vi "Battery_Model_Pulsed_Current.vi"() -> ()   [LabVIEW 2015]
uses:
  <vilib>/Platform/TimedLoop/XDataNode/timing_clust.ctl
  <vilib>/Platform/TimedLoop/XDataNode/nitl_modes.ctl
  <vilib>/Platform/TimedLoop/XDataNode/wakeup.ctl
  Global 1.vi
  <vilib>/Utility/NIReport.llb/NI_report.lvclass
  <vilib>/platform/TimedLoop/XDataNode/XDataNode.xnode
  <instrlib>/Agilent N6700 Series/Agilent N6700 Series.lvlib
  <vilib>/addons/_office/NI_ReportGenerationToolkit.lvlib
  <vilib>/Platform/TimedLoop/XDataNode/XDNodeRunTimeDep.lvlib
panel:
  in  "Stop":bool
  out "Voltage Graph":dbl[](graph)
  in  "Negative Voltage Limit (0.0 volts) 3":dbl format="%^.3e"
  in  "Priority (1: Voltage) 3":i32(ring) items=["Voltage"=1, "Current"=0]
  in  "Positive Voltage Limit  (5.0 V) 3":dbl=5.0 format="%^.3e"
  in  "Channel Name (1) 3":string="4"
  in  "VISA resource name 3":refnum<visa-resource-name>="USB0::0x0957::0x0F07::MY53002228::INSTR"
  in  "report file path 4":path=path "C:/Users/Tulio/Documents/LabView Projects/Battery Model/Battery_Model_Measurements.xlsx"
  out "Current Graph":dbl[](graph)
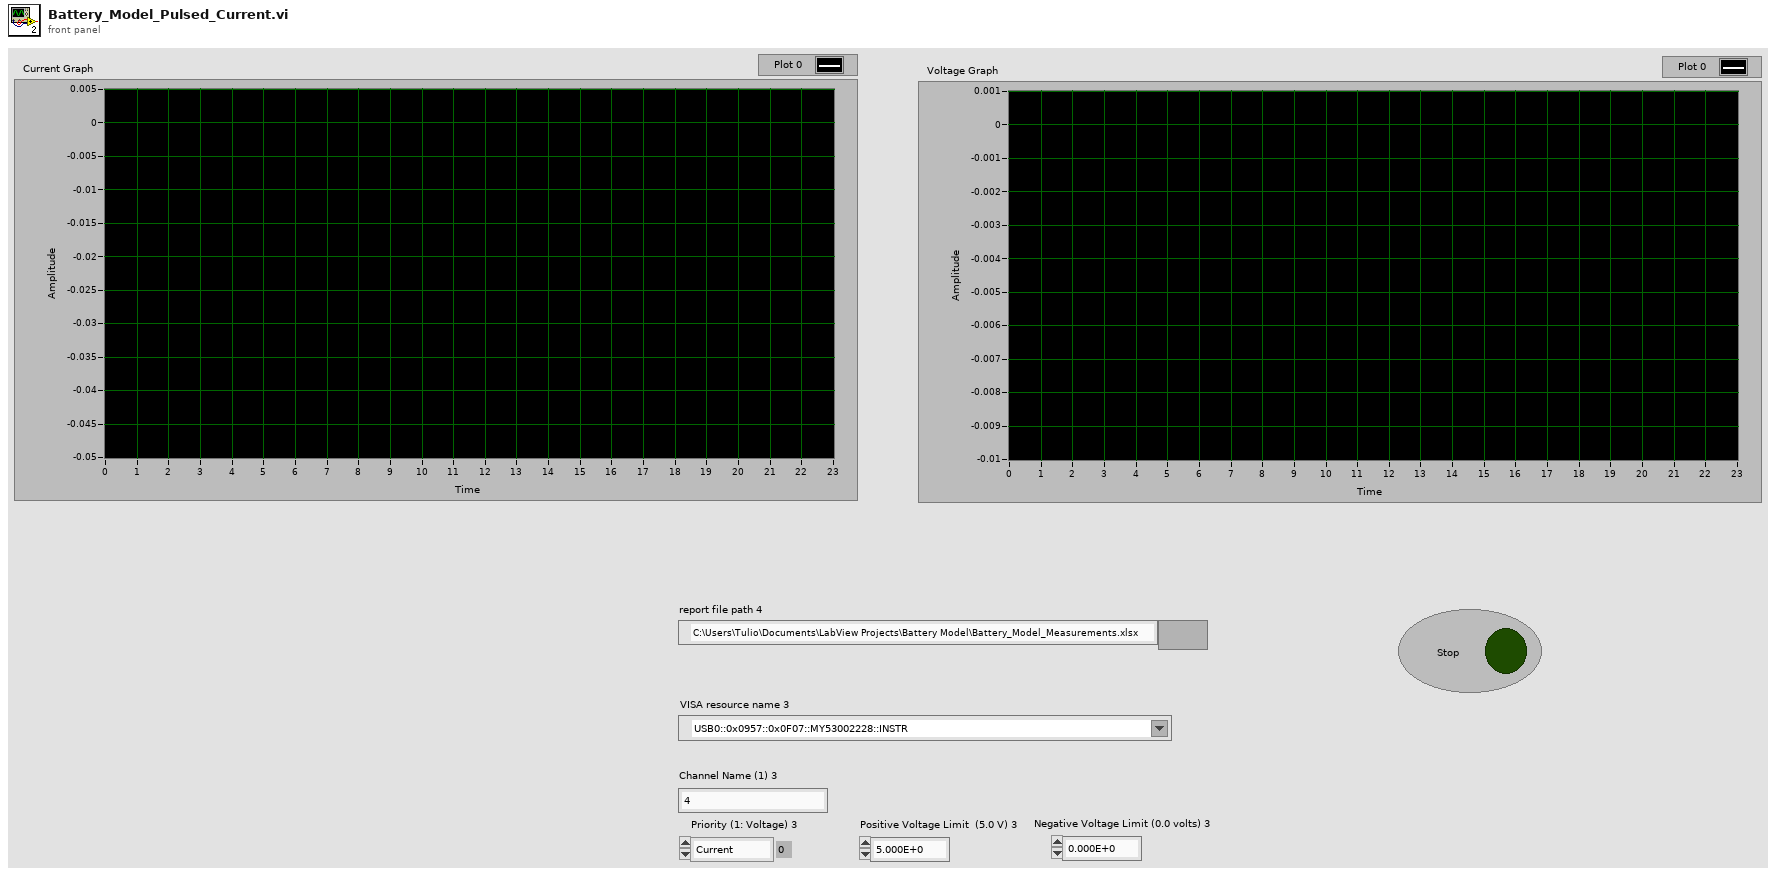
[diagram p1: front panel]
types:
  T1 = enum16{"Standard Report", "HTML", "Word", "Excel"}
  T2 = typedef "XDNodeRunTimeDep.lvlib/timing_clust.ctl" = cluster{"Expected End [f-1]":u64, "Actual End [f-1]":u64, "Finished Late? [f-1]":bool, "Expected End [i-1]":u64, "Actual End [i-1]":u64, "Finished Late? [i-1]":bool, "Expected Start [i]":u64, "Actual Start [i]":u64, "Expected Start [f]":u64, "Actual Start [f]":u64, "Source Name":string, "Structure Name":string, "Period":i64, "Deadline":i64, "Offset":i64, "Start":i64, "Priority":i32, "Timeout":i32, "Mode":T3, "Wakeup Reason":T4, "Error":errorcluster, "Source Type":string, "Secondary Source Type":string, "Global End Time":u64, "Global Start Time":u64, "Frame Duration":u64, "Iteration Duration":u64, "Assigned CPU":i32, "I/O Scan Engine Mode":u32}
  T3 = typedef "XDNodeRunTimeDep.lvlib/nitl_modes.ctl" = enum32{"No Change", "Process missed periods, maintain original phase", "Discard missed periods, maintain original phase", "Process missed periods, ignore original phase", "Discard missed periods, ignore original phase"}
  T4 = typedef "XDNodeRunTimeDep.lvlib/wakeup.ctl" = enum32{"Normal", "Aborted", "Asynchronous wakeup", "Timing source error", "Timed loop error", "Timeout"}
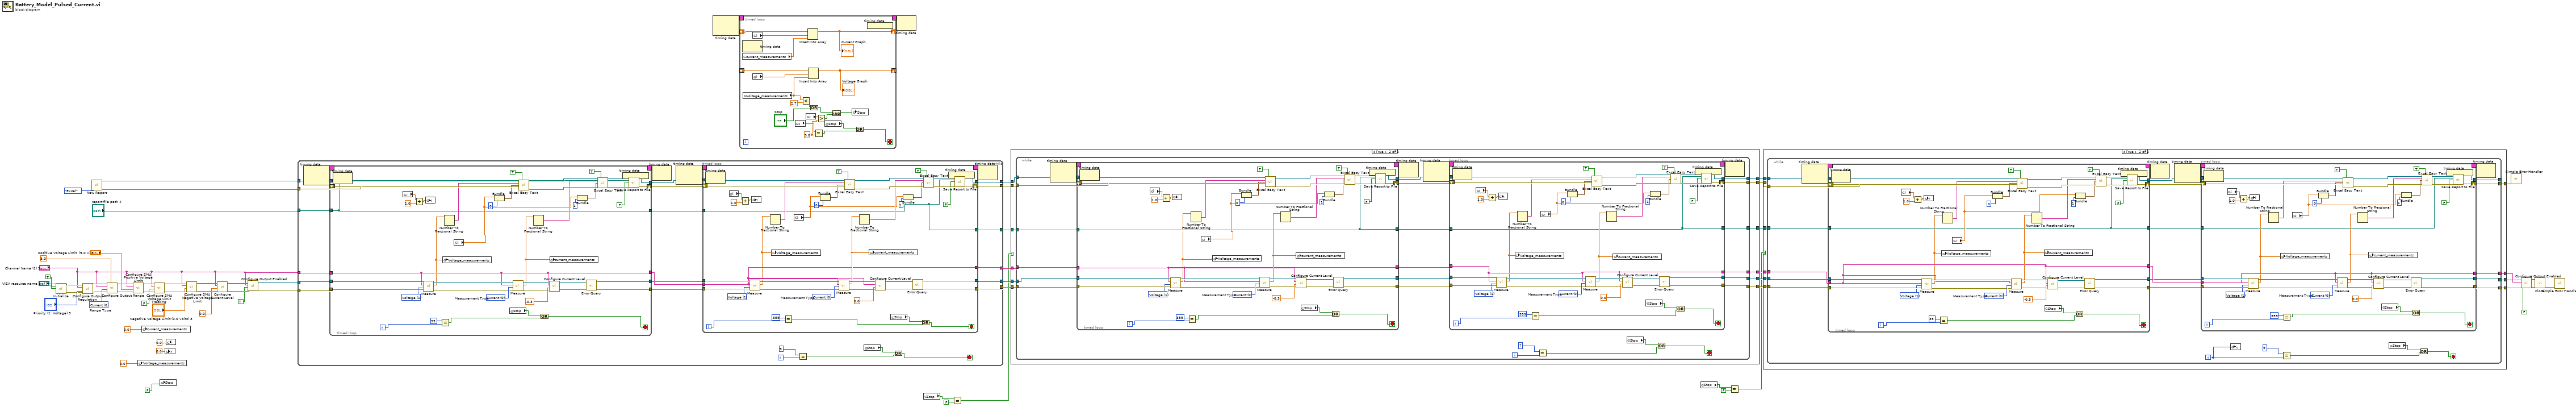
[diagram p0: block diagram]
diagram:
  w49 = TRUE ("Reset? (T: Yes)")
  w48 = 0 items=["Voltage"=1, "Current"=0]  # Range Type
  n1 = call <instrlib>:"Initialize.vi"("VISA resource name"="VISA resource name 3", "ID Query? (T: Yes)"=w49, "Reset? (T: Yes)"=w49) -> ("VISA resource name out"=w38:refnum<visa-resource-name>, "error out"=w37:errorcluster)  [unwired: 11 in]
  n2 = call <instrlib>:"Configure Output Regulation.vi"("VISA resource name"=w38, "Channel Name (1)"="Channel Name (1) 3", "Output Regulation Priority (1: Voltage)"="Priority (1: Voltage) 3", "error in (no error)"=w37) -> ("VISA resource name out"=w50:refnum<visa-resource-name>, "error out"=w51:errorcluster)  [unwired: 10 in]
  n3 = call <vilib>:"New Report.vi"("report type"=T1."Excel") -> ("report out"=w61:refnum<class "NI_report.lvclass">, "error out"=w60:errorcluster)  [unwired: 13 in]
  n4 = call <instrlib>:"Configure Output Range.vi"("Range (0.0)"=3.0, "error in (no error)"=w51, "Range Type (1: Voltage)"=w48, "Channel Name (1)"="Channel Name (1) 3", "VISA resource name"=w50) -> ("error out"=w53:errorcluster, "VISA resource name out"=w52:refnum<visa-resource-name>)  [unwired: 5 in]
  n5 = call <instrlib>:"Configure SMU Positive Voltage Limit.vi"("error in (no error)"=w53, "Positive Voltage Limit (0.0 volts)"="Positive Voltage Limit  (5.0 V) 3", "Channel Name (1)"="Channel Name (1) 3", "VISA resource name"=w52) -> ("error out"=w55:errorcluster, "VISA resource name out"=w54:refnum<visa-resource-name>)  [unwired: 6 in]
  n6 = global write "Global 1.vi" "Voltage_measurements"(0.0 ("Actual_hour")) -> ()
  n7 = global write "Global 1.vi" "current_measurements"(0.0 ("Actual_hour")) -> ()
  n8 = call <instrlib>:"Configure SMU Voltage Limit Tracking.vi"("error in (no error)"=w55, "Enable Voltage Limit Tracking (False)"=FALSE, "Channel Name (1)"="Channel Name (1) 3", "VISA resource name"=w54) -> ("error out"=w42:errorcluster, "VISA resource name out"=w43:refnum<visa-resource-name>)  [unwired: 6 in]
  n9 = global write "Global 1.vi" "Stop"(FALSE ("Stop")) -> ()
  n10 = global write "Global 1.vi" "x"(0.0 ("x")) -> ()
  n11 = global write "Global 1.vi" "i"(0.0 ("Actual_hour")) -> ()
  n12 = call <instrlib>:"Configure SMU Negative Voltage Limit.vi"("error in (no error)"=w42, "Negative Voltage Limit (0.0 volts)"="Negative Voltage Limit (0.0 volts) 3", "Channel Name (1)"="Channel Name (1) 3", "VISA resource name"=w43) -> ("error out"=w39:errorcluster, "VISA resource name out"=w40:refnum<visa-resource-name>)  [unwired: 6 in]
  n13 = call <instrlib>:"Configure Current Level.vi"("error in (no error)"=w39, "Level  (0.0 A)"=0.0, "Channel Name (1)"="Channel Name (1) 3", "VISA resource name"=w40) -> ("error out"=w58:errorcluster, "VISA resource name out"=w59:refnum<visa-resource-name>)  [unwired: 6 in]
  n14 = call <instrlib>:"Configure Output Enabled.vi"("error in (no error)"=w58, "Enable Output (False)"=TRUE, "Channel Name (1)"="Channel Name (1) 3", "VISA resource name"=w59) -> ("error out"=w30:errorcluster, "VISA resource name out"=w31:refnum<visa-resource-name>)  [unwired: 6 in]
  n15 = while {
    tunnel: w31 -> [w89]
    tunnel: w30 -> [w88]
    tunnel: [w68] -> w25
    tunnel: [w70] -> w24
    tunnel: [w72] -> w23
    tunnel: w61 -> [w91]
    tunnel: w60 -> [w90]
    tunnel: "Channel Name (1) 3" -> [w73]
    tunnel: [w78] -> w22
    tunnel: [w77] -> w21
    tunnel: "report file path 4" -> [w76]
    tunnel: [w74] -> w10
    i -> [w80]
    stop <- w66 stop-if-true
    n16 = node-c288() -> (w87:T2)  [unwired: 2 in]
    n17 = timed-loop {
      timing: w87 -> [_]
      timing-out: [_] -> w86
      tunnel: w91 -> [w180]
      tunnel: w73 -> [w143]
      shift-right: [w168] -> w82
      shift-left: w90 -> [w179]
      tunnel: [w148] -> w83
      tunnel: [w143] -> w81
      tunnel: [w144] -> _
      tunnel: w76 -> [w144]
      tunnel: [w144] -> w75
      tunnel: w89 -> [w164]
      tunnel: [w158] -> w71
      tunnel: w88 -> [w163]
      tunnel: [w157] -> w69
      i -> [w146]
      stop <- w139 stop-if-true
      w162 = 1 items=["Current", "Voltage", "Power"] ("Measurement Type (1: Voltage)")
      w181 = 0 items=["Voltage"=1, "Current"=0]  # Measurement Type
      n18 = node-c288() -> ()  [unwired: 1 in, 1 out]
      n19 = global read "Global 1.vi" "i"() -> (w151:dbl)
      n20 = Add(x=w151, y=1.0) -> (x+y=w152:dbl)
      n21 = call <instrlib>:"Measure.vi"("error in (no error)"=w163, "Measurement Type (1: Voltage)"=w162, "Channel Name (1)"=w143, "VISA resource name"=w164) -> ("error out"=w166:errorcluster, "Measurement"=w142:dbl, "VISA resource name out"=w165:refnum<visa-resource-name>)  [unwired: 5 in]
      n22 = global write "Global 1.vi" "i"(w152) -> ()
      n23 = Equal?(x=35, y=w146) -> (x = y?=w141:bool)
      n24 = global write "Global 1.vi" "Voltage_measurements"(w142) -> ()
      n25 = Number To Fractional String(number=w142) -> (F-format string=w161:string)  [unwired: 3 in]
      n26 = global read "Global 1.vi" "i"() -> (w147:dbl)
      n27 = Bundle("i"=w147, "offset (0)"=0) -> (w178:cluster{"i":dbl, "offset (0)":i32})  [unwired: 1 in]
      n28 = global read "Global 1.vi" "Stop"() -> (w140:bool)
      n29 = call <instrlib>:"Measure.vi"("error in (no error)"=w166, "Measurement Type (1: Voltage)"=w181, "Channel Name (1)"=w143, "VISA resource name"=w165) -> ("error out"=w153:errorcluster, "Measurement"=w149:dbl, "VISA resource name out"=w154:refnum<visa-resource-name>)  [unwired: 5 in]
      n30 = call <vilib>:"Excel Easy Text.vi"("report in"=w180, "border? (F)"=TRUE, "text"=w161, "start (-1, -1)"=w178, "error in (no error)"=w179) -> ("report out"=w175:refnum<class "NI_report.lvclass">, "error out"=w176:errorcluster)  [unwired: 6 in, 3 out]
      n31 = Number To Fractional String(number=w149) -> (F-format string=w172:string)  [unwired: 3 in]
      n32 = Or(x=w140, y=w141) -> (x .or. y?=w139:bool)
      n33 = call <instrlib>:"Configure Current Level.vi"("error in (no error)"=w153, "Level  (0.0 A)"=-0.3, "Channel Name (1)"=w143, "VISA resource name"=w154) -> ("error out"=w155:errorcluster, "VISA resource name out"=w156:refnum<visa-resource-name>)  [unwired: 6 in]
      n34 = global write "Global 1.vi" "current_measurements"(w149) -> ()
      n35 = Bundle("i"=w147, "offset (0)"=1) -> (w173:cluster{"i":dbl, "offset (0)":i32})  [unwired: 1 in]
      n36 = call <instrlib>:"Error Query.vi"("VISA resource name"=w156, "error in (no error)"=w155) -> ("VISA resource name out"=w158:refnum<visa-resource-name>, "error out"=w157:errorcluster)  [unwired: 10 in, 2 out]
      n37 = call <vilib>:"Excel Easy Text.vi"("report in"=w175, "border? (F)"=TRUE, "text"=w172, "start (-1, -1)"=w173, "error in (no error)"=w176) -> ("report out"=w170:refnum<class "NI_report.lvclass">, "error out"=w169:errorcluster)  [unwired: 6 in, 3 out]
      n38 = node-c288() -> ()  [unwired: 1 out]
      n39 = call-dynamic "Save Report to File.vi"("report in"=w170, "report file path"=w144, "prompt to replace? (F)"=FALSE, "error in (no error)"=w169) -> ("report out"=w148:refnum<class "NI_report.lvclass">, "error out"=w168:errorcluster)  [unwired: 10 in]
    }
    n40 = node-c288(w86) -> ()  [unwired: 1 out]
    n41 = node-c288() -> (w85:T2)  [unwired: 2 in]
    n42 = timed-loop {
      timing: w85 -> [_]
      timing-out: [_] -> w84
      tunnel: w83 -> [w133]
      tunnel: w81 -> [w96]
      shift-right: [w121] -> w78
      shift-left: w82 -> [w132]
      tunnel: [w98] -> w77
      tunnel: w75 -> [w97]
      tunnel: [w97] -> w74
      tunnel: [w96] -> w72
      tunnel: w71 -> [w117]
      tunnel: [w111] -> w70
      tunnel: w69 -> [w116]
      tunnel: [w110] -> w68
      i -> [w100]
      stop <- w92 stop-if-true
      w115 = 1 items=["Current", "Voltage", "Power"] ("Measurement Type (1: Voltage)")
      w134 = 0 items=["Voltage"=1, "Current"=0]  # Measurement Type
      n43 = node-c288() -> ()  [unwired: 1 in, 1 out]
      n44 = global read "Global 1.vi" "i"() -> (w104:dbl)
      n45 = Add(x=w104, y=1.0) -> (x+y=w105:dbl)
      n46 = call <instrlib>:"Measure.vi"("error in (no error)"=w116, "Measurement Type (1: Voltage)"=w115, "Channel Name (1)"=w96, "VISA resource name"=w117) -> ("error out"=w119:errorcluster, "Measurement"=w95:dbl, "VISA resource name out"=w118:refnum<visa-resource-name>)  [unwired: 5 in]
      n47 = global write "Global 1.vi" "i"(w105) -> ()
      n48 = Number To Fractional String(number=w95) -> (F-format string=w114:string)  [unwired: 3 in]
      n49 = global write "Global 1.vi" "Voltage_measurements"(w95) -> ()
      n50 = Equal?(x=359, y=w100) -> (x = y?=w93:bool)
      n51 = global read "Global 1.vi" "i"() -> (w102:dbl)
      n52 = Bundle("i"=w102, "offset (0)"=0) -> (w131:cluster{"i":dbl, "offset (0)":i32})  [unwired: 1 in]
      n53 = call <instrlib>:"Measure.vi"("error in (no error)"=w119, "Measurement Type (1: Voltage)"=w134, "Channel Name (1)"=w96, "VISA resource name"=w118) -> ("error out"=w106:errorcluster, "Measurement"=w101:dbl, "VISA resource name out"=w107:refnum<visa-resource-name>)  [unwired: 5 in]
      n54 = call <vilib>:"Excel Easy Text.vi"("report in"=w133, "border? (F)"=TRUE, "text"=w114, "start (-1, -1)"=w131, "error in (no error)"=w132) -> ("report out"=w128:refnum<class "NI_report.lvclass">, "error out"=w129:errorcluster)  [unwired: 6 in, 3 out]
      n55 = Number To Fractional String(number=w101) -> (F-format string=w125:string)  [unwired: 3 in]
      n56 = global write "Global 1.vi" "current_measurements"(w101) -> ()
      n57 = call <instrlib>:"Configure Current Level.vi"("error in (no error)"=w106, "Level  (0.0 A)"=0.0, "Channel Name (1)"=w96, "VISA resource name"=w107) -> ("error out"=w108:errorcluster, "VISA resource name out"=w109:refnum<visa-resource-name>)  [unwired: 6 in]
      n58 = global read "Global 1.vi" "Stop"() -> (w94:bool)
      n59 = Bundle("i"=w102, "offset (0)"=1) -> (w126:cluster{"i":dbl, "offset (0)":i32})  [unwired: 1 in]
      n60 = call <instrlib>:"Error Query.vi"("VISA resource name"=w109, "error in (no error)"=w108) -> ("VISA resource name out"=w111:refnum<visa-resource-name>, "error out"=w110:errorcluster)  [unwired: 10 in, 2 out]
      n61 = Or(x=w94, y=w93) -> (x .or. y?=w92:bool)
      n62 = call <vilib>:"Excel Easy Text.vi"("report in"=w128, "border? (F)"=TRUE, "text"=w125, "start (-1, -1)"=w126, "error in (no error)"=w129) -> ("report out"=w123:refnum<class "NI_report.lvclass">, "error out"=w122:errorcluster)  [unwired: 6 in, 3 out]
      n63 = node-c288() -> ()  [unwired: 1 out]
      n64 = call-dynamic "Save Report to File.vi"("report in"=w123, "report file path"=w97, "prompt to replace? (F)"=FALSE, "error in (no error)"=w122) -> ("report out"=w98:refnum<class "NI_report.lvclass">, "error out"=w121:errorcluster)  [unwired: 10 in]
    }
    n65 = Equal?(x=9, y=w80) -> (x = y?=w65:bool)
    n66 = global read "Global 1.vi" "Stop"() -> (w67:bool)
    n67 = Or(x=w67, y=w65) -> (x .or. y?=w66:bool)
    n68 = node-c288(w84) -> ()  [unwired: 1 out]
  }
  n69 = node-c288() -> (w64:T2)  [unwired: 2 in]
  n70 = timed-loop {
    timing: w64 -> [_]
    timing-out: [_] -> w63
    shift-right: [w204] -> _
    shift-left: _ -> [w205]
    shift-right: [w199] -> _
    shift-left: _ -> [w198]
    stop <- w195 stop-if-true
    w186 = 9.0 ("y")
    n71 = node-c288() -> ()  [unwired: 1 in, 1 out]
    n72 = global read "Global 1.vi" "current_measurements"() -> (w202:dbl)
    n73 = global read "Global 1.vi" "Voltage_measurements"() -> (w191:dbl)
    n74 = global read "Global 1.vi" "i"() -> (w203:dbl)
    n75 = global read "Global 1.vi" "i"() -> (w200:dbl)
    n76 = global read "Global 1.vi" "x"() -> (w201:dbl)
    n77 = Less?(x=w191, y=2.7) -> (x < y?=w193:bool)
    n78 = global read "Global 1.vi" "i"() -> (w187:dbl)
    n79 = Insert Into Array(array=w205, index=w203, new element=w202) -> (w204:dbl[])
    "Current Graph" <- w204
    n80 = Insert Into Array(array=w198, index=w200, new element=w191) -> (w199:dbl[])
    "Voltage Graph" <- w199
    n81 = Or(x=w193, y="Stop") -> (x .or. y?=w189:bool)
    n82 = Equal?(x=w201, y=w186) -> (x = y?=w196:bool)
    n83 = Greater?(x=w187, y=w186) -> (0:w188:bool)
    n84 = global read "Global 1.vi" "Stop"() -> (w197:bool)
    n85 = And(x=w189, y=w188) -> (x .and. y?=w190:bool)
    n86 = global write "Global 1.vi" "Stop"(w190) -> ()
    n87 = Or(x=w197, y=w196) -> (x .or. y?=w195:bool)
    n88 = node-c288() -> ()  [unwired: 1 out]
  }
  n89 = node-c288(w63) -> ()  [unwired: 1 out]
  n90 = global read "Global 1.vi" "Stop"() -> (w5:bool)
  n91 = Equal?(x=w5, y=FALSE) -> (x = y?=w6:bool)
  n92 = case shown="True" w6 {
    tunnel: w25 -> [w208 w225]
    tunnel: w24 -> [w209 w224]
    tunnel: w23 -> [w210 w223]
    tunnel: w22 -> [w212 w222]
    tunnel: w21 -> [w213 w221]
    tunnel: [w208 w220] -> w20
    tunnel: [w209 w219] -> w19
    tunnel: [w210 w218] -> w18
    tunnel: [w212 w217] -> w17
    tunnel: [w213 w216] -> w16
    tunnel: w10 -> [w211 w215]
    tunnel: [w211 w214] -> w9
    frame False {
    }
    frame True {
      n93 = while {
        tunnel: w224 -> [w250]
        tunnel: [w230] -> w220
        tunnel: [w231] -> w219
        tunnel: [w233] -> w218
        tunnel: w221 -> [w252]
        tunnel: w222 -> [w251]
        tunnel: w223 -> [w240]
        tunnel: [w239] -> w217
        tunnel: w225 -> [w238]
        tunnel: [w237] -> w216
        tunnel: w215 -> [w236]
        tunnel: [w234] -> w214
        i -> [w242]
        stop <- w227 stop-if-true
        n94 = node-c288() -> (w249:T2)  [unwired: 2 in]
        n95 = timed-loop {
          timing: w249 -> [_]
          timing-out: [_] -> w248
          tunnel: w252 -> [w341]
          tunnel: w240 -> [w308]
          shift-right: [w329] -> w244
          shift-left: w251 -> [w340]
          tunnel: [w309] -> w245
          tunnel: [w308] -> w243
          tunnel: w236 -> [w304]
          tunnel: [w304] -> w235
          tunnel: w250 -> [w325]
          tunnel: [w319] -> w229
          tunnel: w238 -> [w324]
          tunnel: [w318] -> w232
          i -> [w306]
          stop <- w300 stop-if-true
          w323 = 1 items=["Current", "Voltage", "Power"] ("Measurement Type (1: Voltage)")
          w342 = 0 items=["Voltage"=1, "Current"=0]  # Measurement Type
          n96 = node-c288() -> ()  [unwired: 1 in, 1 out]
          n97 = global read "Global 1.vi" "i"() -> (w312:dbl)
          n98 = Add(x=w312, y=1.0) -> (x+y=w313:dbl)
          n99 = call <instrlib>:"Measure.vi"("error in (no error)"=w324, "Measurement Type (1: Voltage)"=w323, "Channel Name (1)"=w308, "VISA resource name"=w325) -> ("error out"=w327:errorcluster, "Measurement"=w303:dbl, "VISA resource name out"=w326:refnum<visa-resource-name>)  [unwired: 5 in]
          n100 = global write "Global 1.vi" "i"(w313) -> ()
          n101 = Equal?(x=359, y=w306) -> (x = y?=w301:bool)
          n102 = Number To Fractional String(number=w303) -> (F-format string=w322:string)  [unwired: 3 in]
          n103 = global read "Global 1.vi" "i"() -> (w307:dbl)
          n104 = global write "Global 1.vi" "Voltage_measurements"(w303) -> ()
          n105 = Bundle("i"=w307, "offset (0)"=0) -> (w339:cluster{"i":dbl, "offset (0)":i32})  [unwired: 1 in]
          n106 = call <instrlib>:"Measure.vi"("error in (no error)"=w327, "Measurement Type (1: Voltage)"=w342, "Channel Name (1)"=w308, "VISA resource name"=w326) -> ("error out"=w314:errorcluster, "Measurement"=w310:dbl, "VISA resource name out"=w315:refnum<visa-resource-name>)  [unwired: 5 in]
          n107 = call <vilib>:"Excel Easy Text.vi"("report in"=w341, "border? (F)"=TRUE, "text"=w322, "start (-1, -1)"=w339, "error in (no error)"=w340) -> ("report out"=w336:refnum<class "NI_report.lvclass">, "error out"=w337:errorcluster)  [unwired: 6 in, 3 out]
          n108 = Number To Fractional String(number=w310) -> (F-format string=w333:string)  [unwired: 3 in]
          n109 = global write "Global 1.vi" "current_measurements"(w310) -> ()
          n110 = call <instrlib>:"Configure Current Level.vi"("error in (no error)"=w314, "Level  (0.0 A)"=-0.3, "Channel Name (1)"=w308, "VISA resource name"=w315) -> ("error out"=w316:errorcluster, "VISA resource name out"=w317:refnum<visa-resource-name>)  [unwired: 6 in]
          n111 = global read "Global 1.vi" "Stop"() -> (w302:bool)
          n112 = Bundle("i"=w307, "offset (0)"=1) -> (w334:cluster{"i":dbl, "offset (0)":i32})  [unwired: 1 in]
          n113 = Or(x=w302, y=w301) -> (x .or. y?=w300:bool)
          n114 = call <instrlib>:"Error Query.vi"("VISA resource name"=w317, "error in (no error)"=w316) -> ("VISA resource name out"=w319:refnum<visa-resource-name>, "error out"=w318:errorcluster)  [unwired: 10 in, 2 out]
          n115 = call <vilib>:"Excel Easy Text.vi"("report in"=w336, "border? (F)"=TRUE, "text"=w333, "start (-1, -1)"=w334, "error in (no error)"=w337) -> ("report out"=w331:refnum<class "NI_report.lvclass">, "error out"=w330:errorcluster)  [unwired: 6 in, 3 out]
          n116 = node-c288() -> ()  [unwired: 1 out]
          n117 = call-dynamic "Save Report to File.vi"("report in"=w331, "report file path"=w304, "prompt to replace? (F)"=FALSE, "error in (no error)"=w330) -> ("report out"=w309:refnum<class "NI_report.lvclass">, "error out"=w329:errorcluster)  [unwired: 10 in]
        }
        n118 = node-c288(w248) -> ()  [unwired: 1 out]
        n119 = node-c288() -> (w247:T2)  [unwired: 2 in]
        n120 = timed-loop {
          timing: w247 -> [_]
          timing-out: [_] -> w246
          tunnel: w245 -> [w294]
          tunnel: w243 -> [w257]
          shift-right: [w282] -> w239
          shift-left: w244 -> [w293]
          tunnel: [w259] -> w237
          tunnel: w235 -> [w258]
          tunnel: [w258] -> w234
          tunnel: [w257] -> w233
          tunnel: w232 -> [w277]
          tunnel: [w271] -> w230
          tunnel: w229 -> [w278]
          tunnel: [w272] -> w231
          i -> [w261]
          stop <- w253 stop-if-true
          w276 = 1 items=["Current", "Voltage", "Power"] ("Measurement Type (1: Voltage)")
          w295 = 0 items=["Voltage"=1, "Current"=0]  # Measurement Type
          n121 = node-c288() -> ()  [unwired: 1 in, 1 out]
          n122 = global read "Global 1.vi" "i"() -> (w265:dbl)
          n123 = Add(x=w265, y=1.0) -> (x+y=w266:dbl)
          n124 = call <instrlib>:"Measure.vi"("error in (no error)"=w277, "Measurement Type (1: Voltage)"=w276, "Channel Name (1)"=w257, "VISA resource name"=w278) -> ("error out"=w280:errorcluster, "Measurement"=w256:dbl, "VISA resource name out"=w279:refnum<visa-resource-name>)  [unwired: 5 in]
          n125 = global write "Global 1.vi" "i"(w266) -> ()
          n126 = global write "Global 1.vi" "Voltage_measurements"(w256) -> ()
          n127 = Number To Fractional String(number=w256) -> (F-format string=w275:string)  [unwired: 3 in]
          n128 = Equal?(x=359, y=w261) -> (x = y?=w254:bool)
          n129 = global read "Global 1.vi" "i"() -> (w263:dbl)
          n130 = Bundle("i"=w263, "offset (0)"=0) -> (w292:cluster{"i":dbl, "offset (0)":i32})  [unwired: 1 in]
          n131 = call <instrlib>:"Measure.vi"("error in (no error)"=w280, "Measurement Type (1: Voltage)"=w295, "Channel Name (1)"=w257, "VISA resource name"=w279) -> ("error out"=w267:errorcluster, "Measurement"=w262:dbl, "VISA resource name out"=w268:refnum<visa-resource-name>)  [unwired: 5 in]
          n132 = call <vilib>:"Excel Easy Text.vi"("report in"=w294, "border? (F)"=TRUE, "text"=w275, "start (-1, -1)"=w292, "error in (no error)"=w293) -> ("report out"=w289:refnum<class "NI_report.lvclass">, "error out"=w290:errorcluster)  [unwired: 6 in, 3 out]
          n133 = Number To Fractional String(number=w262) -> (F-format string=w286:string)  [unwired: 3 in]
          n134 = global write "Global 1.vi" "current_measurements"(w262) -> ()
          n135 = call <instrlib>:"Configure Current Level.vi"("error in (no error)"=w267, "Level  (0.0 A)"=0.0, "Channel Name (1)"=w257, "VISA resource name"=w268) -> ("error out"=w269:errorcluster, "VISA resource name out"=w270:refnum<visa-resource-name>)  [unwired: 6 in]
          n136 = global read "Global 1.vi" "Stop"() -> (w255:bool)
          n137 = Bundle("i"=w263, "offset (0)"=1) -> (w287:cluster{"i":dbl, "offset (0)":i32})  [unwired: 1 in]
          n138 = call <instrlib>:"Error Query.vi"("VISA resource name"=w270, "error in (no error)"=w269) -> ("VISA resource name out"=w272:refnum<visa-resource-name>, "error out"=w271:errorcluster)  [unwired: 10 in, 2 out]
          n139 = call <vilib>:"Excel Easy Text.vi"("report in"=w289, "border? (F)"=TRUE, "text"=w286, "start (-1, -1)"=w287, "error in (no error)"=w290) -> ("report out"=w284:refnum<class "NI_report.lvclass">, "error out"=w283:errorcluster)  [unwired: 6 in, 3 out]
          n140 = Or(x=w255, y=w254) -> (x .or. y?=w253:bool)
          n141 = node-c288() -> ()  [unwired: 1 out]
          n142 = call-dynamic "Save Report to File.vi"("report in"=w284, "report file path"=w258, "prompt to replace? (F)"=FALSE, "error in (no error)"=w283) -> ("report out"=w259:refnum<class "NI_report.lvclass">, "error out"=w282:errorcluster)  [unwired: 10 in]
        }
        n143 = Equal?(x=7, y=w242) -> (x = y?=w226:bool)
        n144 = global read "Global 1.vi" "Stop"() -> (w228:bool)
        n145 = Or(x=w228, y=w226) -> (x .or. y?=w227:bool)
        n146 = node-c288(w246) -> ()  [unwired: 1 out]
      }
    }
  }
  n147 = global read "Global 1.vi" "Stop"() -> (w3:bool)
  n148 = Equal?(x=w3, y=FALSE) -> (x = y?=w1:bool)
  n149 = case shown="True" w1 {
    tunnel: w20 -> [w347 w360]
    tunnel: w19 -> [w348 w359]
    tunnel: w18 -> [w349 w358]
    tunnel: w17 -> [w350 w357]
    tunnel: w16 -> [_ w356]
    tunnel: [w347 w355] -> w15
    tunnel: [w349 w354] -> w14
    tunnel: [w350 w353] -> w13
    tunnel: [w348 w352] -> w12
    tunnel: w9 -> [_ w351]
    frame False {
    }
    frame True {
      n150 = while {
        tunnel: w359 -> [w384]
        tunnel: [w364] -> w355
        tunnel: [w367] -> w352
        tunnel: [w368] -> w354
        tunnel: w356 -> [w386]
        tunnel: w357 -> [w385]
        tunnel: w358 -> [w369]
        tunnel: [w375] -> w353
        tunnel: [w374] -> _
        tunnel: w360 -> [w373]
        tunnel: w351 -> [w371]
        i -> [w372]
        stop <- w362 stop-if-true
        n151 = node-c288() -> (w383:T2)  [unwired: 2 in]
        n152 = timed-loop {
          timing: w383 -> [_]
          timing-out: [_] -> w382
          tunnel: w386 -> [w475]
          tunnel: w369 -> [w442]
          shift-right: [w463] -> w378
          shift-left: w385 -> [w474]
          tunnel: [w443] -> w379
          tunnel: [w442] -> w377
          tunnel: w371 -> [w438]
          tunnel: [w438] -> w370
          tunnel: w384 -> [w459]
          tunnel: [w453] -> w366
          tunnel: w373 -> [w458]
          tunnel: [w452] -> w365
          i -> [w440]
          stop <- w434 stop-if-true
          w457 = 1 items=["Current", "Voltage", "Power"] ("Measurement Type (1: Voltage)")
          w476 = 0 items=["Voltage"=1, "Current"=0]  # Measurement Type
          n153 = node-c288() -> ()  [unwired: 1 in, 1 out]
          n154 = global read "Global 1.vi" "i"() -> (w446:dbl)
          n155 = Add(x=w446, y=1.0) -> (x+y=w447:dbl)
          n156 = call <instrlib>:"Measure.vi"("error in (no error)"=w458, "Measurement Type (1: Voltage)"=w457, "Channel Name (1)"=w442, "VISA resource name"=w459) -> ("error out"=w461:errorcluster, "Measurement"=w437:dbl, "VISA resource name out"=w460:refnum<visa-resource-name>)  [unwired: 5 in]
          n157 = global write "Global 1.vi" "i"(w447) -> ()
          n158 = Equal?(x=35, y=w440) -> (x = y?=w435:bool)
          n159 = global write "Global 1.vi" "Voltage_measurements"(w437) -> ()
          n160 = Number To Fractional String(number=w437) -> (F-format string=w456:string)  [unwired: 3 in]
          n161 = global read "Global 1.vi" "i"() -> (w441:dbl)
          n162 = Bundle("i"=w441, "offset (0)"=0) -> (w473:cluster{"i":dbl, "offset (0)":i32})  [unwired: 1 in]
          n163 = call <instrlib>:"Measure.vi"("error in (no error)"=w461, "Measurement Type (1: Voltage)"=w476, "Channel Name (1)"=w442, "VISA resource name"=w460) -> ("error out"=w448:errorcluster, "Measurement"=w444:dbl, "VISA resource name out"=w449:refnum<visa-resource-name>)  [unwired: 5 in]
          n164 = call <vilib>:"Excel Easy Text.vi"("report in"=w475, "border? (F)"=TRUE, "text"=w456, "start (-1, -1)"=w473, "error in (no error)"=w474) -> ("report out"=w470:refnum<class "NI_report.lvclass">, "error out"=w471:errorcluster)  [unwired: 6 in, 3 out]
          n165 = Number To Fractional String(number=w444) -> (F-format string=w467:string)  [unwired: 3 in]
          n166 = global write "Global 1.vi" "current_measurements"(w444) -> ()
          n167 = global read "Global 1.vi" "Stop"() -> (w436:bool)
          n168 = call <instrlib>:"Configure Current Level.vi"("error in (no error)"=w448, "Level  (0.0 A)"=-0.3, "Channel Name (1)"=w442, "VISA resource name"=w449) -> ("error out"=w450:errorcluster, "VISA resource name out"=w451:refnum<visa-resource-name>)  [unwired: 6 in]
          n169 = Or(x=w436, y=w435) -> (x .or. y?=w434:bool)
          n170 = Bundle("i"=w441, "offset (0)"=1) -> (w468:cluster{"i":dbl, "offset (0)":i32})  [unwired: 1 in]
          n171 = call <instrlib>:"Error Query.vi"("VISA resource name"=w451, "error in (no error)"=w450) -> ("VISA resource name out"=w453:refnum<visa-resource-name>, "error out"=w452:errorcluster)  [unwired: 10 in, 2 out]
          n172 = call <vilib>:"Excel Easy Text.vi"("report in"=w470, "border? (F)"=TRUE, "text"=w467, "start (-1, -1)"=w468, "error in (no error)"=w471) -> ("report out"=w465:refnum<class "NI_report.lvclass">, "error out"=w464:errorcluster)  [unwired: 6 in, 3 out]
          n173 = node-c288() -> ()  [unwired: 1 out]
          n174 = call-dynamic "Save Report to File.vi"("report in"=w465, "report file path"=w438, "prompt to replace? (F)"=FALSE, "error in (no error)"=w464) -> ("report out"=w443:refnum<class "NI_report.lvclass">, "error out"=w463:errorcluster)  [unwired: 10 in]
        }
        n175 = node-c288(w382) -> ()  [unwired: 1 out]
        n176 = node-c288() -> (w381:T2)  [unwired: 2 in]
        n177 = timed-loop {
          timing: w381 -> [_]
          timing-out: [_] -> w380
          tunnel: w379 -> [w428]
          tunnel: w377 -> [w391]
          shift-right: [w416] -> w375
          shift-left: w378 -> [w427]
          tunnel: [w393] -> w374
          tunnel: w370 -> [w392]
          tunnel: [w391] -> w368
          tunnel: w365 -> [w411]
          tunnel: [w405] -> w364
          tunnel: w366 -> [w412]
          tunnel: [w406] -> w367
          i -> [w395]
          stop <- w387 stop-if-true
          w410 = 1 items=["Current", "Voltage", "Power"] ("Measurement Type (1: Voltage)")
          w429 = 0 items=["Voltage"=1, "Current"=0]  # Measurement Type
          n178 = node-c288() -> ()  [unwired: 1 in, 1 out]
          n179 = global read "Global 1.vi" "i"() -> (w399:dbl)
          n180 = Add(x=w399, y=1.0) -> (x+y=w400:dbl)
          n181 = call <instrlib>:"Measure.vi"("error in (no error)"=w411, "Measurement Type (1: Voltage)"=w410, "Channel Name (1)"=w391, "VISA resource name"=w412) -> ("error out"=w414:errorcluster, "Measurement"=w390:dbl, "VISA resource name out"=w413:refnum<visa-resource-name>)  [unwired: 5 in]
          n182 = global write "Global 1.vi" "i"(w400) -> ()
          n183 = Number To Fractional String(number=w390) -> (F-format string=w409:string)  [unwired: 3 in]
          n184 = global write "Global 1.vi" "Voltage_measurements"(w390) -> ()
          n185 = Equal?(x=359, y=w395) -> (x = y?=w388:bool)
          n186 = global read "Global 1.vi" "i"() -> (w397:dbl)
          n187 = Bundle("i"=w397, "offset (0)"=0) -> (w426:cluster{"i":dbl, "offset (0)":i32})  [unwired: 1 in]
          n188 = call <instrlib>:"Measure.vi"("error in (no error)"=w414, "Measurement Type (1: Voltage)"=w429, "Channel Name (1)"=w391, "VISA resource name"=w413) -> ("error out"=w401:errorcluster, "Measurement"=w396:dbl, "VISA resource name out"=w402:refnum<visa-resource-name>)  [unwired: 5 in]
          n189 = call <vilib>:"Excel Easy Text.vi"("report in"=w428, "border? (F)"=TRUE, "text"=w409, "start (-1, -1)"=w426, "error in (no error)"=w427) -> ("report out"=w423:refnum<class "NI_report.lvclass">, "error out"=w424:errorcluster)  [unwired: 6 in, 3 out]
          n190 = Number To Fractional String(number=w396) -> (F-format string=w420:string)  [unwired: 3 in]
          n191 = global write "Global 1.vi" "current_measurements"(w396) -> ()
          n192 = call <instrlib>:"Configure Current Level.vi"("error in (no error)"=w401, "Level  (0.0 A)"=0.0, "Channel Name (1)"=w391, "VISA resource name"=w402) -> ("error out"=w403:errorcluster, "VISA resource name out"=w404:refnum<visa-resource-name>)  [unwired: 6 in]
          n193 = global read "Global 1.vi" "Stop"() -> (w389:bool)
          n194 = Bundle("i"=w397, "offset (0)"=1) -> (w421:cluster{"i":dbl, "offset (0)":i32})  [unwired: 1 in]
          n195 = call <instrlib>:"Error Query.vi"("VISA resource name"=w404, "error in (no error)"=w403) -> ("VISA resource name out"=w406:refnum<visa-resource-name>, "error out"=w405:errorcluster)  [unwired: 10 in, 2 out]
          n196 = Or(x=w389, y=w388) -> (x .or. y?=w387:bool)
          n197 = call <vilib>:"Excel Easy Text.vi"("report in"=w423, "border? (F)"=TRUE, "text"=w420, "start (-1, -1)"=w421, "error in (no error)"=w424) -> ("report out"=w418:refnum<class "NI_report.lvclass">, "error out"=w417:errorcluster)  [unwired: 6 in, 3 out]
          n198 = node-c288() -> ()  [unwired: 1 out]
          n199 = call-dynamic "Save Report to File.vi"("report in"=w418, "report file path"=w392, "prompt to replace? (F)"=FALSE, "error in (no error)"=w417) -> ("report out"=w393:refnum<class "NI_report.lvclass">, "error out"=w416:errorcluster)  [unwired: 10 in]
        }
        n200 = global write "Global 1.vi" "x"(w372) -> ()
        n201 = Equal?(x=9, y=w372) -> (x = y?=w361:bool)
        n202 = global read "Global 1.vi" "Stop"() -> (w363:bool)
        n203 = Or(x=w363, y=w361) -> (x .or. y?=w362:bool)
        n204 = node-c288(w380) -> ()  [unwired: 1 out]
      }
    }
  }
  n205 = call <vilib>:"Simple Error Handler.vi"("error in (no error)"=w13) -> ()  [unwired: 1 in, 8 out]
  n206 = call <instrlib>:"Configure Output Enabled.vi"("error in (no error)"=w15, "Enable Output (False)"=FALSE, "Channel Name (1)"=w14, "VISA resource name"=w12) -> ("error out"=w28:errorcluster, "VISA resource name out"=w27:refnum<visa-resource-name>)  [unwired: 6 in]
  n207 = call <instrlib>:"Close.vi"("VISA resource name"=w27, "error in (no error)"=w28) -> ("error out"=w26:errorcluster)  [unwired: 13 in]
  n208 = call <vilib>:"Simple Error Handler.vi"("error in (no error)"=w26) -> ()  [unwired: 4 in, 5 out]
